vi "Data_Get_Spectrum_Number.vi"(8 "error in (no error)":errorcluster, 10 "Setup":string, 11 "Path of the Day":path) -> (0 "error out":errorcluster caption="sortie d'erreur", 2 "Last Spectrum Number":string, 3 "Next Spectrum Number":string)   [LabVIEW 2017]
doc: "This VI returns the next spectrum prefix available, with the naming convention yyyy_mm_dd_xxx.\nxxx is the spectrum number."
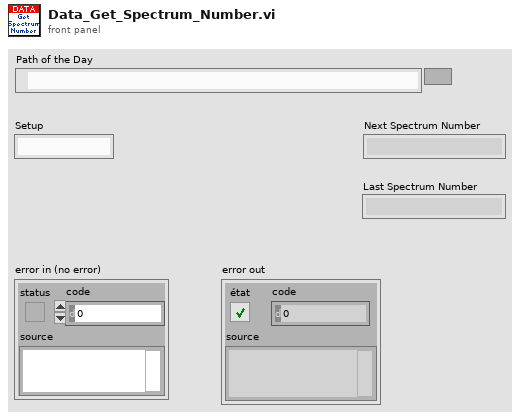
[diagram p1: front panel]
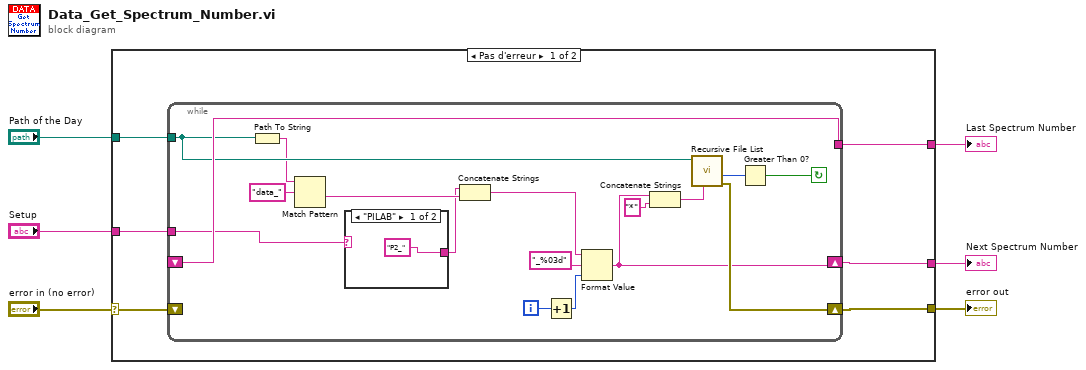
[diagram p0: block diagram]
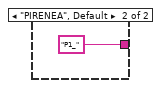
[diagram p2: hidden frame]
diagram:
  n1 = case shown="Pas d'erreur" "error in (no error)" {
    selector: "error in (no error)" -> [w11 w32]
    tunnel: "Path of the Day" -> [w12 _]
    tunnel: [w10 w32] -> w4
    tunnel: [w9 _] -> w3
    tunnel: [w8 _] -> w2
    tunnel: "Setup" -> [w7 _]
    frame No Error {
      n2 = while {
        tunnel: w12 -> [w19]
        shift-right: [w28] -> w10
        shift-left: w11 -> [_]
        shift-right: [w21] -> w9
        shift-left: _ -> [w20]
        tunnel: [w20] -> w8
        tunnel: w7 -> [w14]
        i -> [w27]
        stop <- w24 continue-if-true
        n3 = Path To String(path=w19) -> (string=w18:string)
        n4 = Match Pattern(string=w18, regular expression="data_" ("expression régulière")) -> (after substring=w16:string)  [unwired: 1 in, 3 out]
        n5 = case shown="\"PILAB\"" w14 {
          tunnel: ["P2_" "P1_"] -> w13
          frame "PILAB" {
          }
          frame "PIRENEA", Default {
          }
        }
        n6 = Concatenate Strings(w13, w16) -> (w15:string)
        n7 = Increment(x=w27) -> (x+1=w26:i32)
        n8 = Format Value(string ("")=w15, format string="_%03d" ("chaîne de format"), value (0)=w26) -> (output string=w21:string)
        n9 = Concatenate Strings(w21, "*" ("chaîne")) -> (w22:string)
        n10 = call <vilib>:"Recursive File List.vi"("pattern"=w22, "Folder Path"=w19) -> ("error out"=w28:errorcluster, "Number of Files"=w25:i32)  [unwired: 5 in, 3 out]
        n11 = Greater Than 0?(x=w25) -> (x > 0?=w24:bool)
      }
    }
    frame Error {
    }
  }
  "error out" <- w4
  "Next Spectrum Number" <- w3
  "Last Spectrum Number" <- w2
